vi "LVClass_DataServer SetSlopes.vi"(0 "DataServer in":refnum<class "DataServer.lvclass">, 5 "name":string, 7 "HasoSlopes in":refnum<class "HasoSlopes.lvclass">, 11 "error in (no error)":errorcluster) -> (4 "DataServer out":refnum<class "DataServer.lvclass">, 8 "HasoSlopes (dup)":refnum<class "HasoSlopes.lvclass">, 15 "error out":errorcluster)   [LabVIEW 2020, in "DataServer.lvclass"]
doc: "Set the slopes to be send by TCP connection.\n\n--------------------------------------------------------------------------------\n\n<B>serverIn </B> : Server object.\n<B>serverOut </B> : Server object.\n<B>hasoslopes </B> : HasoSlopes object.\n<B>ErrorIn </B> : Error\n<B>ErrorOut </B> : Error\n\n--------------------------------------------------------------------------------"
uses:
  DataServer.lvclass
  HasoSlopes.lvclass
  DataServer.lvclass/DataServer.ctl
  LVClass_HasoSlopes Read HasoSlopes _ property.vi
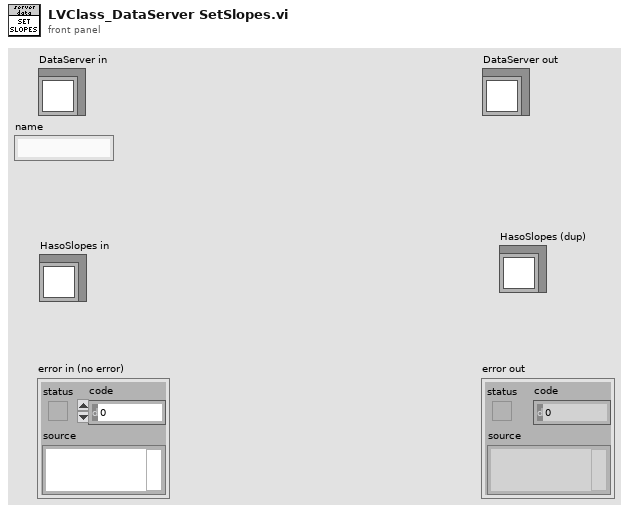
[diagram p1: front panel]
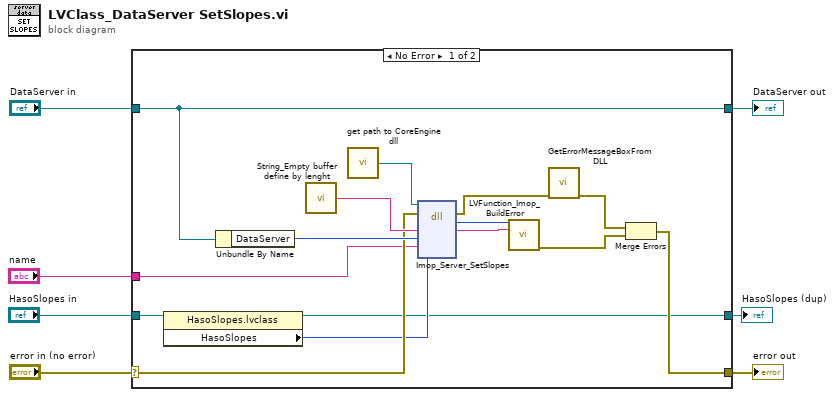
[diagram p0: block diagram]
diagram:
  n1 = case shown="No Error" "error in (no error)" {
    selector: "error in (no error)" -> [w13 w25]
    tunnel: [w12 w25] -> w6
    tunnel: [w14 w24] -> w4
    tunnel: "DataServer in" -> [w14 w24]
    tunnel: "HasoSlopes in" -> [w11 w23]
    tunnel: [w9 w23] -> w2
    tunnel: "name" -> [w8 _]
    frame No Error {
      n2 = property class="HasoSlopes.lvclass"(reference=w11) -> (reference out=w9:refnum<class "HasoSlopes.lvclass">, "HasoSlopes"=w10:i32)  [unwired: 1 in, 1 out]
      n3 = Unbundle By Name(w14) -> ("DataServer"=w20:i32)
      n4 = call "String_Empty buffer define by lenght.vi"() -> ("Empty buffer"=w17:string)  [unwired: 1 in]
      n5 = call "get path to CoreEngine dll.vi"() -> ("path to c_interface_vc100.dll"=w18:path)  [unwired: 12 in, 3 out]
      n6 = dll-call lib="D:/soft/HASO_v3/SVN_trunk/ImOpCoreEngine4_LV2011/DLLs/c_interface_vc100.dll" fn="Imop_Server_SetSlopes"(path in=w18, error in=w13, "message"=w17, "server"=w20, "name"=w8, "data"=w10) -> (error out=w19:errorcluster, "return type"=w15:i32, "message"=w16:string)  [unwired: 4 in, 1 out]
      n7 = call "LVFunction_Imop_BuildError.vi"("code"=w15, "String to Prepend to source (\"\")"=w16) -> ("error out"=w22:errorcluster)  [unwired: 13 in]
      n8 = call "GetErrorMessageBoxFromDLL.vi"("error IN"=w19) -> ("error OUT"=w21:errorcluster)  [unwired: 10 in]
      n9 = Merge Errors(w21, w22) -> (w12:errorcluster)
    }
    frame Error {
    }
  }
  "error out" <- w6
  "DataServer out" <- w4
  "HasoSlopes (dup)" <- w2
